vi "Stop Core.vi"(10 "final error code":i32, 11 "Analyze Actor in":refnum<class "Analyze Actor.lvclass">) -> (3 "Analyze Actor out":refnum<class "Analyze Actor.lvclass">)   [LabVIEW 2020, in "Analyze Actor.lvlib" / "Analyze Actor.lvclass"]
doc: "(<B>Filename</B>: Actor Framework.lvlib:Actor.lvclass:Stop Core.vi)\n\nDefines what the actor does before it stops. Use the <B>final error code</B> input to determine whether the actor shut down in response to an error.\n\nBy default, this method passes the Stop message along to all auto-stop nested actors. A descendant class may override this method to define additional behavior, such as shutting down any processes the actor initiated in its override of the Actor Core method."
uses:
  Analyze Actor.lvclass
  Analyze Actor.lvclass/Analyze Actor.ctl
  <vilib>/ActorFramework/Actor/Actor.lvclass
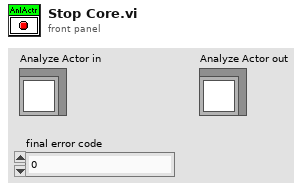
[diagram p1: front panel]
types:
  T1 = typedef "IMAQ Image.ctl" = refnum<image>
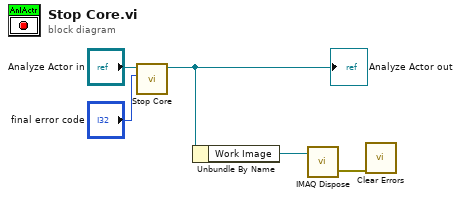
[diagram p0: block diagram]
diagram:
  n1 = call-parent "Stop Core.vi"("final error code"="final error code", "Actor in"="Analyze Actor in") -> ("Actor out"=w3:refnum<class "Analyze Actor.lvclass">)  [unwired: 9 in]
  "Analyze Actor out" <- w3
  n2 = Unbundle By Name(w3) -> ("Work Image"=w2:T1)
  n3 = call "IMAQ Dispose"("Image"=w2) -> ("error out"=w1:errorcluster)  [unwired: 5 in]
  n4 = call <vilib>:"Clear Errors.vi"("error in (no error)"=w1) -> ()  [unwired: 5 in, 2 out]
